vi "fgv_save-info.vi"(7 "cmd":T2, 11 "save info":T1) -> (3 "save info 2":T1)   [LabVIEW 2019]
uses:
  _ctrl/rw.ctl
  result-path.ctl
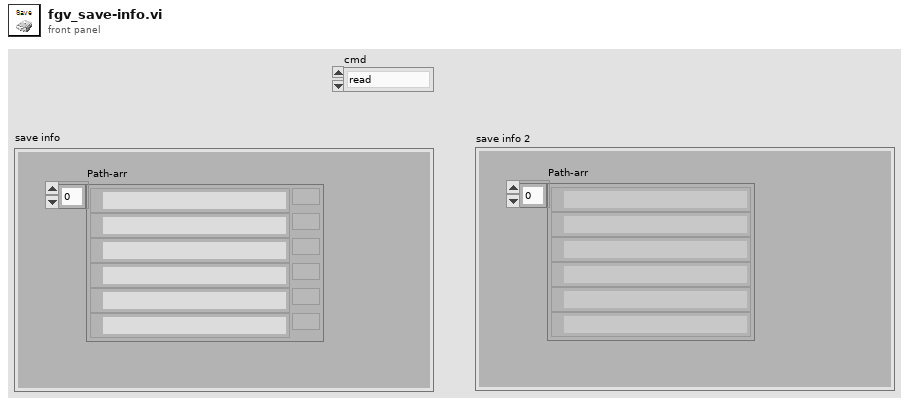
[diagram p1: front panel]
types:
  T1 = typedef "result-path.ctl" = cluster{"Path-arr":path[]}
  T2 = typedef "rw.ctl" = enum16{"read", "write"}
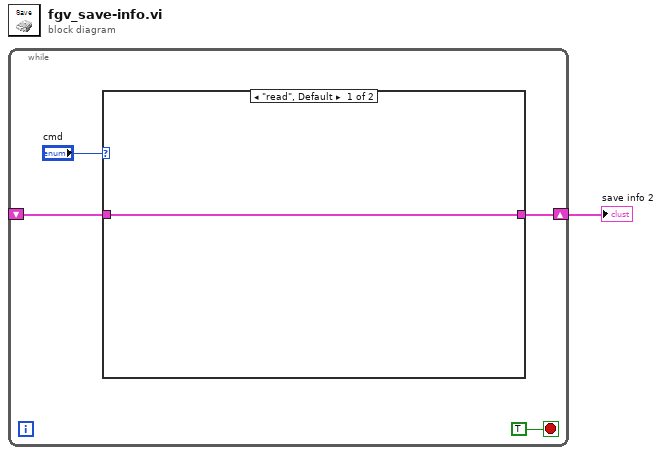
[diagram p0: block diagram]
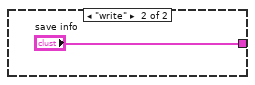
[diagram p2: hidden frame]
diagram:
  n1 = while {
    shift-right: [w3] -> w1
    shift-left: _ -> [w2]
    stop <- TRUE stop-if-true
    n2 = case shown="\"read\", Default" "cmd" {
      tunnel: [w6 "save info"] -> w3
      tunnel: w2 -> [w6 _]
      frame "read", Default {
      }
      frame "write" {
      }
    }
  }
  "save info 2" <- w1
